vi "Path to String Path.vi"(1 "Path":path) -> (0 "String":string)   [LabVIEW 2020, in "feature_detection.lvlib" / "Text Recognizer.lvclass"]
uses:
  Text Recognizer.lvclass
  Text Recognizer.lvclass/Text Recognizer.ctl
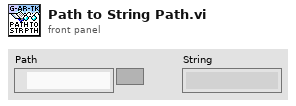
[diagram p1: front panel]
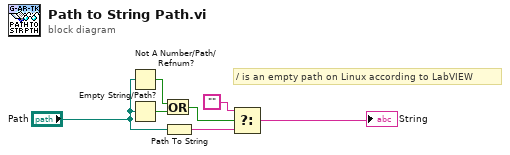
[diagram p0: block diagram]
diagram:
  # "/ is an empty path on Linux according to LabVIEW"
  n1 = Not A Number/Path/Refnum?(number/path/refnum="Path") -> (NaN/Path/Refnum?=w1:bool)
  n2 = Empty String/Path?(string/path="Path") -> (empty?=w2:bool)
  n3 = Or(x=w1, y=w2) -> (x .or. y?=w3:bool)
  n4 = Path To String(path="Path") -> (string=w6:string)
  n5 = Select(t="", s=w3, f=w6) -> (s? t:f=→"String":string)
